vi "Main.vi"(10 "Productos Subpanel":refnum<vi>, 11 "Module Admin":refnum<class "Delacor_lib_QMH_Module Admin.lvclass">) -> ()   [LabVIEW 2020, in "Productos.lvlib"]
doc: "This template is based off of the Queued Message Handler design pattern and the Queued Message Handler project template that ships with LabVIEW.\n\nThe main difference is that the queue is private to this module and communication between modules is performed via Broadcast and Request events.\n\nRequest events are wrapped in public API methods and are handled in the Event Handling Loop (EHL) of this VI. Any module can register for Broadcast events sent by this module. The EHL generates messages based on user interface actions.\n\nThe Message Handling Loop (MHL) processes messages generated by the EHL, or by other messages. The messages are string values, so new messages can be added easily to the Message Cases case structure in the MHL. Each message cluster can also provide an optional value for Message Data, which is a variant that can be converted to whatever message-specific data is required.\n_____\nBased on Delacor QMH Project Template 5.0.0.82."
uses:
  Productos.lvlib
  <vilib>/Delacor/Delacor QMH/Libraries/Module Admin_class/Delacor_lib_QMH_Module Admin.lvclass
  Module Data--cluster.ctl
  Stop Argument--cluster.ctl
  <vilib>/Delacor/Delacor QMH/Libraries/Message Queue_class/Delacor_lib_QMH_Message Queue.lvclass/Delacor_lib_QMH_Message Queue.ctl
  <vilib>/Delacor/Delacor QMH/Libraries/Module Admin_class/Delacor_lib_QMH_Module Admin.lvclass/Delacor_lib_QMH_Module Admin.ctl
  <vilib>/Delacor/Delacor QMH/Libraries/Message Queue_class/Delacor_lib_QMH_Enqueue Message (Single).vi
  <vilib>/Delacor/Delacor QMH/Libraries/Module Admin_class/Delacor_lib_QMH_Get External Launch.vi
  <vilib>/Utility/error.llb/Error Cluster From Error Code.vi
  <vilib>/ErrorRing/Error Ring.xnode
  <vilib>/Delacor/Delacor QMH/Libraries/Message Queue_class/Delacor_lib_QMH_Message Queue.lvclass
panel:
  out "Status":string
  out "subarray":string[](array[string])
  in  "stop":bool
  in  "Products":i32(listbox)
  out "error out":errorcluster
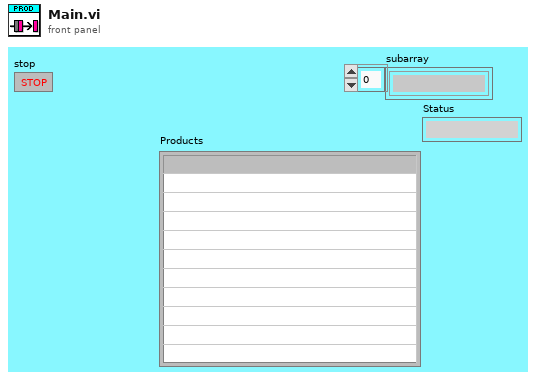
[diagram p1: front panel]
types:
  T1 = typedef "Productos.lvlib/Request Events--cluster.ctl" = cluster{"Stop Module":refnum<user-event>, "Show Panel":refnum<user-event>, "Hide Panel":refnum<user-event>, "Get Module Execution Status":refnum<user-event>, "Show Diagram":refnum<user-event>}
  T2 = typedef "Productos.lvlib/Module Data--cluster.ctl" = cluster{"Status":string}
  T3 = enum32{"invalid lock state", "Not Locked", "Locked (No Password)", "Password-protected"}
  T4 = typedef "Productos.lvlib/Stop Argument--cluster.ctl" = cluster{"Origin":string, "Exit via Stop Module Req?":bool, "Wait for Module to stop?":bool}
  T5 = enum32{"Invalid", "Standard", "Closed", "Hidden", "Minimized", "Maximized"}
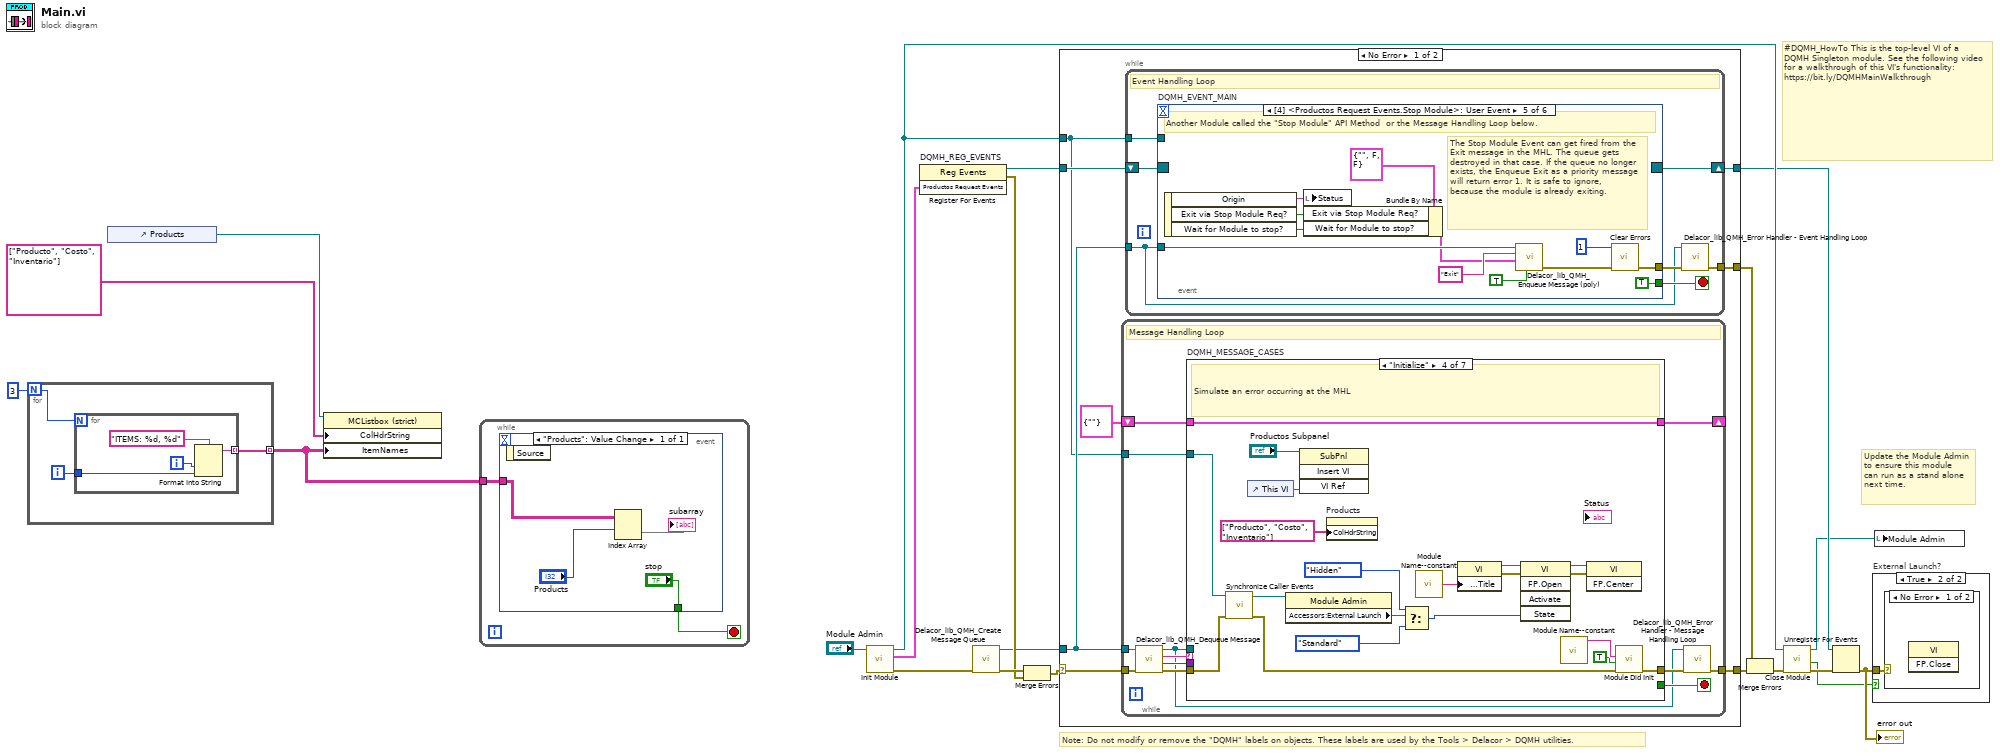
[diagram p0: block diagram]
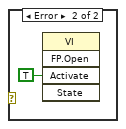
[diagram p3: hidden frame]
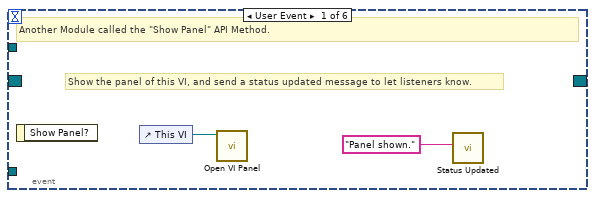
[diagram p4: hidden frame]
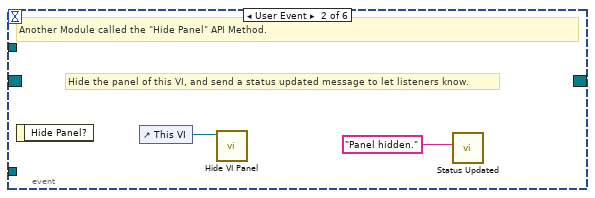
[diagram p5: hidden frame]
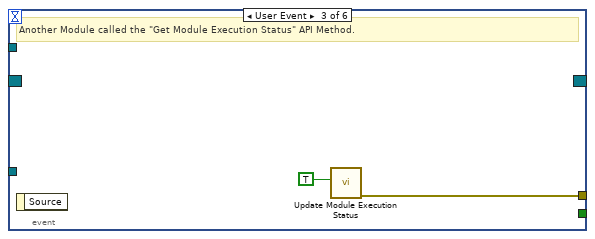
[diagram p6: hidden frame]
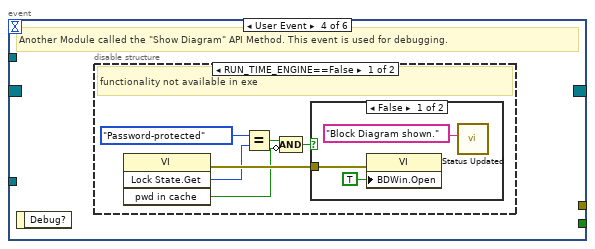
[diagram p7: hidden frame]
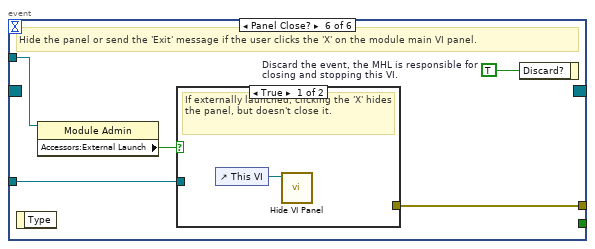
[diagram p10: hidden frame]
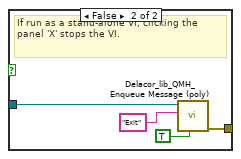
[diagram p11: hidden frame]
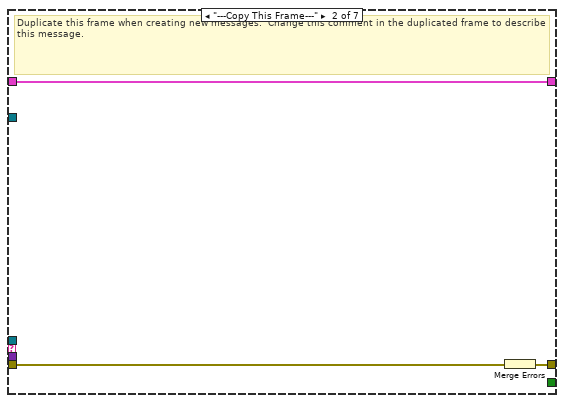
[diagram p13: hidden frame]
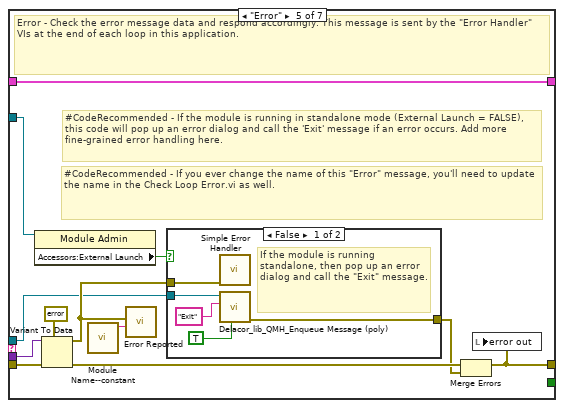
[diagram p15: hidden frame]
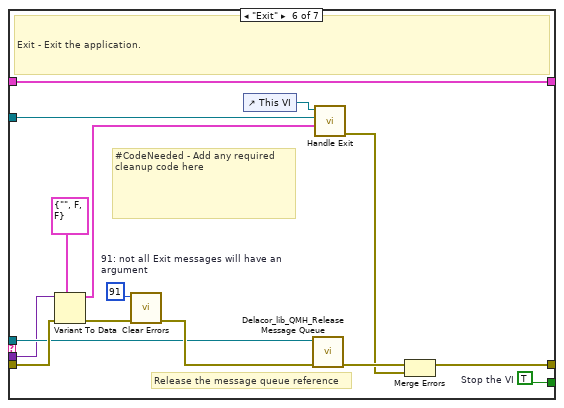
[diagram p17: hidden frame]
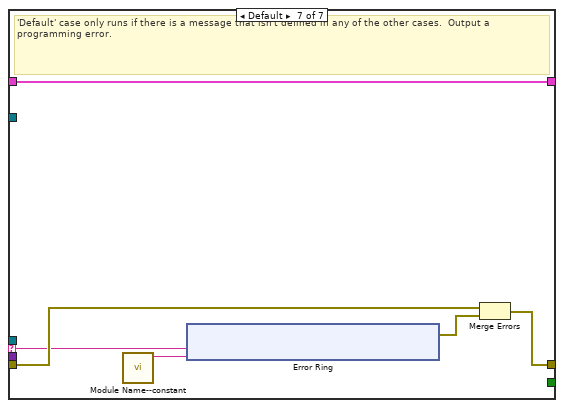
[diagram p18: hidden frame]
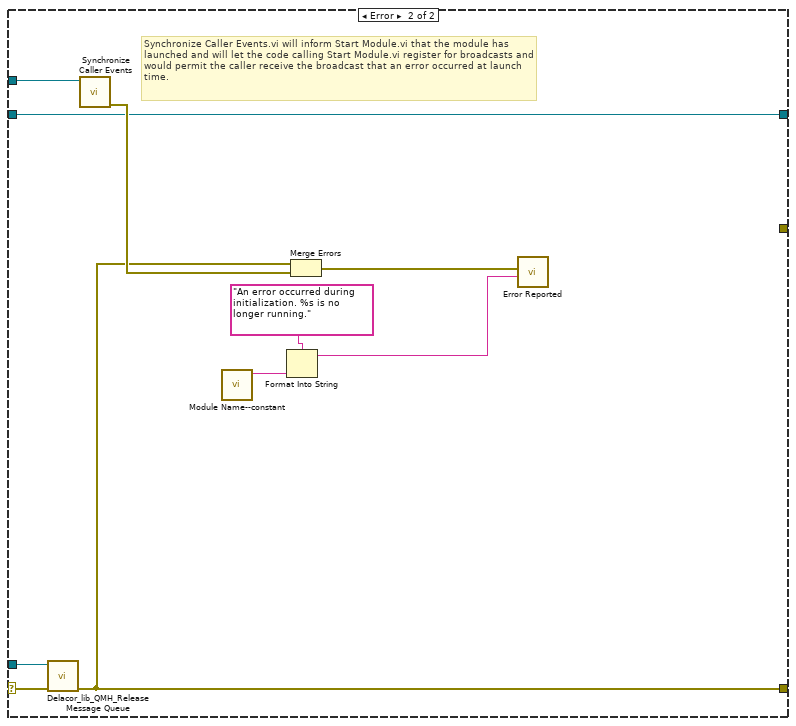
[diagram p19: hidden frame]
diagram:
  # "#DQMH_HowTo This is the top-level VI of a DQMH Singleton module. See the following video for a walkthrough of this VI's functionality: https://bit.ly/DQMHMainWalkthrough"
  # "Note: Do not modify or remove the \"DQMH\" labels on objects. These labels are used by the Tools > Delacor > DQMH utilities."
  # "Update the Module Admin to ensure this module can run as a stand alone next time."
  n1 = for {
    N: 3 -> [w24]
    tunnel: [w23] -> w1 mode=indexing
    i -> [w22]
    n2 = for {
      N: w24 -> [_]
      tunnel: [w27] -> w23 mode=indexing
      tunnel: w22 -> [w25]
      i -> [w28]
      n3 = Format Into String(format string="ITEMS: %d, %d", w28, w25) -> (resulting string=w27:string)  [unwired: 2 in, 1 out]
    }
  }
  n4 = control-ref of="Products"() -> (w4:refnum<vi>)
  n5 = property class="MCListbox (strict)"(reference=w4, "ColHdrString"=string[] ["Producto", "Costo", "Inventario"] ("Column Header Strings[]"), "ItemNames"=w1) -> ()  [unwired: 1 in, 2 out]
  n6 = while {
    tunnel: w1 -> [w30]
    stop <- w29 stop-if-true
    n7 = event shown="[0] \"Products\": Value Change" {
      selector: _ -> [_]
      dyn-events: _ -> [_]
      timeout: _ -> [_]
      tunnel: w30 -> [w34]
      tunnel: ["stop"] -> w29
      event "Products": Value Change {
        n8 = event-data() -> ()  [unwired: 1 in, 1 out]
        n9 = Index Array(array=w34, index (row)="Products") -> (element=→"subarray":string[])  [unwired: 1 in]
      }
    }
  }
  n10 = call "Init Module.vi"("Singleton Module Admin in"="Module Admin") -> ("error out"=w20:errorcluster, "Productos Request Events"=w9:T1, "Singleton Module Admin out"=w12:refnum<class "Delacor_lib_QMH_Module Admin.lvclass">)  [unwired: 8 in]
  n11 = register-events "DQMH_REG_EVENTS"(w9) -> (reference out=w10:refnum<event-registration>, error out=w13:errorcluster)  [unwired: 2 in]
  n12 = call <vilib>:"Delacor_lib_QMH_Create Message Queue.vi"("error in (no error)"=w20) -> ("error out"=w15:errorcluster, "Message Queue"=w8:refnum<class "Delacor_lib_QMH_Message Queue.lvclass">)  [unwired: 9 in]
  n13 = Merge Errors(w15, w13) -> (w14:errorcluster)
  n14 = case shown="No Error" w14 {
    selector: w14 -> [w40 w174]
    tunnel: [w42 w173] -> w21
    tunnel: [w39 w179] -> w11
    tunnel: w10 -> [w37 w179]
    tunnel: w8 -> [w36 w172]
    tunnel: [w41 _] -> w18
    tunnel: w12 -> [w35 w175]
    frame No Error {
      n15 = while {
        tunnel: w36 -> [w89]
        shift-right: [w93] -> _
        shift-left: T2 {"Status"=""} ("Data Cluster") -> [w94]
        tunnel: w40 -> [w97]
        tunnel: [w95] -> w42
        tunnel: w35 -> [w87]
        stop <- w92 stop-if-true
        # "Message Handling Loop"
        n16 = call-dynamic "Delacor_lib_QMH_Dequeue Message.vi"("error in (no error)"=w97, "Message Queue in"=w89) -> ("error out"=w96:errorcluster, "Message Data"=w90:variant, "Message"=w91:string, "Message Queue out"=w88:refnum<class "Delacor_lib_QMH_Message Queue.lvclass">)  [unwired: 6 in]
        n17 = case "DQMH_MESSAGE_CASES" shown="\"Initialize\"" w91 {
          selector: w91 -> [_ _ _ _ _ _ w159]
          tunnel: w88 -> [_ _ _ _ w129 w151 _]
          tunnel: w96 -> [w100 w103 w105 w124 w136 w157 w161]
          tunnel: [w100 w102 w105 w109 w132 w154 w162] -> w98
          tunnel: w94 -> [w99 w101 w104 w125 w131 w150 w160]
          tunnel: [w99 w101 w104 w125 w131 w150 w160] -> w93
          tunnel: [_ _ _ _ _ w149 _] -> w92
          tunnel: w90 -> [_ _ _ _ w130 w148 _]
          tunnel: w87 -> [_ _ _ w123 w128 w143 _]
          frame "--- Module Specific ---" {
            # "Separator -- The following cases handle messages specific to this Module."
          }
          frame "---Copy This Frame---" {
            # "Duplicate this frame when creating new messages.  Change this comment in the duplicated frame to describe this message."
            n18 = Merge Errors(w103) -> (w102:errorcluster)
          }
          frame "--- Exit and Error Handling---" {
            # "Separator - The following cases handle errors and exit messages."
          }
          frame "Initialize" {
            # "Simulate an error occurring at the MHL"
            n19 = call "Synchronize Caller Events.vi"("error in (no error)"=w124, "Singleton Module Admin in"=w123) -> ("error out"=w110:errorcluster, "Singleton Module Admin out"=w122:refnum<class "Delacor_lib_QMH_Module Admin.lvclass">)  [unwired: 8 in]
            n20 = control-ref of="This VI"() -> (w115:refnum<vi>)
            n21 = property class="Module Admin"(reference=w122) -> ("Accessors:External Launch"=w121:bool)  [unwired: 1 in, 2 out]
            n22 = invoke class="SubPnl" method="Insert VI"(reference="Productos Subpanel", "VI Ref"=w115) -> ()  [unwired: 2 in, 4 out]
            n23 = property on="Products" class="MCListbox (strict)"("ColHdrString"=string[] ["Producto", "Costo", "Inventario"] ("Column Header Strings[]")) -> ()  [unwired: 2 in, 2 out]
            n24 = Select(t=T5."Hidden" ("State"), s=w121, f=T5."Standard" ("State")) -> (s? t:f=w113:T5)
            n25 = call "Module Name--constant.vi"() -> ("Module Name"=w114:string)  [unwired: 11 in]
            n26 = property class="VI"("Front Panel.Title"=w114) -> (reference out=w118:refnum<vi>, error out=w120:errorcluster)  [unwired: 2 in]
            n27 = invoke class="VI" method="FP.Open"(reference=w118, error in=w120, "State"=w113) -> (reference out=w117:refnum<vi>, error out=w119:errorcluster)  [unwired: 2 in, 3 out]
            n28 = call "Module Name--constant.vi"() -> ("Module Name"=w108:string)  [unwired: 11 in]
            n29 = invoke class="VI" method="FP.Center"(reference=w117, error in=w119) -> ()  [unwired: 1 in, 3 out]
            n30 = call "Module Did Init.vi"("error in (no error)"=w110, "Initialized?"=TRUE, "Origin"=w108) -> ("error out"=w109:errorcluster)  [unwired: 8 in]
          }
          frame "Error" {
            # "#CodeRecommended - If you ever change the name of this \"Error\" message, you'll need to update the name in the Check Loop Error.vi as well."
            # "#CodeRecommended - If the module is running in standalone mode (External Launch = FALSE), this code will pop up an error dialog and call the 'Exit' message if an error occurs. Add more fine-grained error handling here."
            # "Error - Check the error message data and respond accordingly. This message is sent by the \"Error Handler\" VIs at the end of each loop in this application."
            n31 = property class="Module Admin"(reference=w128) -> ("Accessors:External Launch"=w127:bool)  [unwired: 1 in, 2 out]
            n32 = Variant To Data(error in=w136, type=errorcluster {"status"=FALSE, "code"=0, "source"=""} ("error constant"), Variant=w130) -> (data=w137:errorcluster, error out=w134:errorcluster)
            n33 = call "Module Name--constant.vi"() -> ("Module Name"=w126:string)  [unwired: 11 in]
            n34 = call "Error Reported.vi"("Additional Information"=w126, "Error"=w137) -> ()  [unwired: 9 in, 1 out]
            n35 = case shown="False" w127 {
              tunnel: [w142 _] -> w133
              tunnel: w129 -> [w140 _]
              tunnel: w137 -> [w141 _]
              frame False {
                # "If the module is running standalone, then pop up an error dialog and call the \"Exit\" message."
                n36 = call <vilib>:"Simple Error Handler.vi"("error in (no error)"=w141) -> ()  [unwired: 4 in, 5 out]
                n37 = call-poly <vilib>:"Delacor_lib_QMH_Enqueue Message (poly).vi"("Priority Message? (F)"=TRUE, "Message"="Exit", "Message Queue in"=w140) -> ("error out"=w142:errorcluster)  [unwired: 7 in, 1 out]
              }
              frame True {
                # "If the module was launched externally, calling the Error Reported broadcast VI is the only action performed by the \"Error\" message. The module's caller can then process the error appropriately."
              }
            }
            n38 = Merge Errors(w134, w133) -> (w132:errorcluster)
            n39 = local write "error out"(w132) -> ()
          }
          frame "Exit" {
            w147 = 91  # 91: not all Exit messages will have an argument
            w149 = TRUE  # Stop the VI
            # "Release the message queue reference"
            # "#CodeNeeded - Add any required cleanup code here"
            # "Exit - Exit the application."
            n40 = Variant To Data(error in=w157, type=T4 {"Origin"="", "Exit via Stop Module Req?"=FALSE, "Wait for Module to stop?"=FALSE} ("Stop Argument"), Variant=w148) -> (data=w145:T4, error out=w153:errorcluster)
            n41 = call <vilib>:"Clear Errors.vi"("error in (no error)"=w153, "specific error code to clear (0: all)"=w147) -> ("error out"=w156:errorcluster)  [unwired: 4 in, 1 out]
            n42 = control-ref of="This VI"() -> (w144:refnum<vi>)
            n43 = call-dynamic "Delacor_lib_QMH_Release Message Queue.vi"("error in (no error)"=w156, "Message Queue"=w151) -> ("error out"=w155:errorcluster)  [unwired: 9 in]
            n44 = call "Handle Exit.vi"("Stop Argument"=w145, "Admin in"=w143, "VI reference"=w144) -> ("error out"=w152:errorcluster)  [unwired: 7 in, 1 out]
            n45 = Merge Errors(w155, w152) -> (w154:errorcluster)
          }
          frame Default {
            # "'Default' case only runs if there is a message that isn't defined in any of the other cases.  Output a programming error."
            n46 = call "Module Name--constant.vi"() -> ("Module Name"=w158:string)  [unwired: 11 in]
            n47 = xnode "Error Ring"("parameter 0"=w159, "parameter 1"=w158) -> ("error out"=w163:errorcluster)
            n48 = Merge Errors(w161, w163) -> (w162:errorcluster)
          }
        }
        n49 = call-dynamic "Delacor_lib_QMH_Error Handler - Message Handling Loop.vi"("error in (no error)"=w98, "Message Queue in"=w88) -> ("dup error in"=w95:errorcluster)  [unwired: 8 in, 1 out]
      }
      n50 = while {
        tunnel: w36 -> [w43]
        shift-right: [w46] -> w39
        shift-left: w37 -> [w47]
        tunnel: [w48] -> w41
        tunnel: w35 -> [w44]
        stop <- w45 stop-if-true
        # "Event Handling Loop"
        n51 = event "DQMH_EVENT_MAIN" shown="[4] <Productos Request Events.Stop Module>: User Event" {
          selector: w47 -> [_ _ _ _ _ _]
          dyn-events: [_ _ _ _ _ _] -> w46
          timeout: _ -> [_ _ _ _ _ _]
          tunnel: [_ _ _ _ TRUE ("Discard?") _] -> w45
          tunnel: w43 -> [_ _ _ _ w72 w79]
          tunnel: [_ _ w55 _ w75 w81] -> w49
          tunnel: w44 -> [_ _ _ _ _ w78]
          event User Event {
            # "Show the panel of this VI, and send a status updated message to let listeners know."
            # "Another Module called the \"Show Panel\" API Method."
            n52 = event-data() -> ()  [unwired: 1 in, 1 out]
            n53 = control-ref of="This VI"() -> (w51:refnum<vi>)
            n54 = call "Open VI Panel.vi"("VI"=w51) -> ()  [unwired: 10 in, 1 out]
            n55 = call "Status Updated.vi"("Status"="Panel shown." ("format string")) -> ()  [unwired: 10 in, 1 out]
          }
          event User Event {
            # "Hide the panel of this VI, and send a status updated message to let listeners know."
            # "Another Module called the \"Hide Panel\" API Method."
            n56 = event-data() -> ()  [unwired: 1 in, 1 out]
            n57 = control-ref of="This VI"() -> (w53:refnum<vi>)
            n58 = call "Hide VI Panel.vi"("VI"=w53) -> ()  [unwired: 10 in, 1 out]
            n59 = call "Status Updated.vi"("Status"="Panel hidden." ("format string")) -> ()  [unwired: 10 in, 1 out]
          }
          event User Event {
            # "Another Module called the \"Get Module Execution Status\" API Method."
            n60 = event-data() -> ()  [unwired: 1 in, 1 out]
            n61 = call "Update Module Execution Status.vi"("Running?"=TRUE) -> ("error out"=w55:errorcluster)  [unwired: 10 in]
          }
          event User Event {
            # "Another Module called the \"Show Diagram\" API Method. This event is used for debugging."
            n62 = event-data() -> ()  [unwired: 1 in, 1 out]
            n63 = disable-structure shown="RUN_TIME_ENGINE==False" {
              frame condition #0 (active) {
                # "functionality not available in exe"
                n64 = invoke class="VI" method="Lock State.Get"() -> (error out=w61:errorcluster, "Get Lock State"=w60:T3, "pwd in cache"=w57:bool)  [unwired: 4 in, 1 out]
                n65 = Equal?(x=T3."Password-protected", y=w60) -> (x = y?=w58:bool)
                n66 = Compound Arithmetic op=AND(w58, invert w57) -> (w56:bool)
                n67 = case shown="False" w56 {
                  tunnel: w61 -> [w64 _]
                  frame False {
                    n68 = property class="VI"(error in=w64, "BDWin.Open"=TRUE ("Block Diagram Window:Open")) -> ()  [unwired: 1 in, 2 out]
                    n69 = call "Status Updated.vi"("Status"="Block Diagram shown." ("format string")) -> ()  [unwired: 10 in, 1 out]
                  }
                  frame True {
                    # "Password-protected VI, and the password is not in the cache. Do not show the diagram."
                  }
                }
              }
              frame condition #1 {
              }
            }
          }
          event User Event {
            # "The Stop Module Event can get fired from the Exit message in the MHL. The queue gets destroyed in that case. If the queue no longer exists, the Enqueue Exit as a priority message will return error 1. It is safe to ignore, because the module is already exiting."
            # "Another Module called the \"Stop Module\" API Method  or the Message Handling Loop below."
            n70 = event-data() -> ("Origin"=w65:string, "Exit via Stop Module Req?"=w68:bool, "Wait for Module to stop?"=w67:bool)  [unwired: 1 in]
            n71 = local write "Status"(w65) -> ()
            n72 = Bundle By Name(cluster=T4 {"Origin"="", "Exit via Stop Module Req?"=FALSE, "Wait for Module to stop?"=FALSE} ("Stop Argument"), "Exit via Stop Module Req?"=w68, "Wait for Module to stop?"=w67) -> (w66:T4)
            n73 = call-poly <vilib>:"Delacor_lib_QMH_Enqueue Message (poly).vi"("Priority Message? (F)"=TRUE, "Message Data"=w66, "Message"="Exit", "Message Queue in"=w72) -> ("error out"=w76:errorcluster)  [unwired: 6 in, 1 out]
            n74 = call <vilib>:"Clear Errors.vi"("error in (no error)"=w76, "specific error code to clear (0: all)"=1) -> ("error out"=w75:errorcluster)  [unwired: 4 in, 1 out]
          }
          event Panel Close? {
            w80 = TRUE  # Discard the event, the MHL is responsible for closing and stopping this VI.
            # "Hide the panel or send the 'Exit' message if the user clicks the 'X' on the module main VI panel."
            n75 = event-data() -> ()  [unwired: 1 in, 1 out]
            n76 = property class="Module Admin"(reference=w78) -> ("Accessors:External Launch"=w77:bool)  [unwired: 1 in, 2 out]
            n77 = case shown="True" w77 {
              tunnel: w79 -> [_ w85]
              tunnel: [_ w86] -> w81
              frame True {
                # "If externally launched, clicking the 'X' hides the panel, but doesn't close it."
                n78 = control-ref of="This VI"() -> (w82:refnum<vi>)
                n79 = call "Hide VI Panel.vi"("VI"=w82) -> ()  [unwired: 10 in, 1 out]
              }
              frame False {
                # "If run as a stand-alone VI, clicking the panel 'X' stops the VI."
                n80 = call-poly <vilib>:"Delacor_lib_QMH_Enqueue Message (poly).vi"("Priority Message? (F)"=TRUE, "Message"="Exit", "Message Queue in"=w85) -> ("error out"=w86:errorcluster)  [unwired: 7 in, 1 out]
              }
            }
            n81 = event-data("Discard?"=w80) -> ()  [unwired: 1 in, 1 out]
          }
        }
        n82 = call-dynamic "Delacor_lib_QMH_Error Handler - Event Handling Loop.vi"("error in (no error)"=w49, "Message Queue in"=w43) -> ("dup error in"=w48:errorcluster)  [unwired: 8 in, 1 out]
      }
    }
    frame Error {
      # "Synchronize Caller Events.vi will inform Start Module.vi that the module has launched and will let the code calling Start Module.vi register for broadcasts and would permit the caller receive the broadcast that an error occurred at launch time."
      n83 = call-dynamic "Delacor_lib_QMH_Release Message Queue.vi"("error in (no error)"=w174, "Message Queue"=w172) -> ("error out"=w173:errorcluster)  [unwired: 9 in]
      n84 = call "Synchronize Caller Events.vi"("Singleton Module Admin in"=w175) -> ("error out"=w180:errorcluster)  [unwired: 9 in, 1 out]
      n85 = call "Module Name--constant.vi"() -> ("Module Name"=w178:string)  [unwired: 11 in]
      n86 = Format Into String(format string="An error occurred during initialization. %s is no longer running.", w178) -> (resulting string=w176:string)  [unwired: 2 in, 1 out]
      n87 = Merge Errors(w173, w180) -> (w181:errorcluster)
      n88 = call "Error Reported.vi"("Additional Information"=w176, "Error"=w181) -> ()  [unwired: 9 in, 1 out]
    }
  }
  n89 = Merge Errors(w18, w21) -> (w17:errorcluster)
  n90 = call "Close Module.vi"("error in (no error)"=w17, "Module Admin in"=w12) -> ("error out"=w19:errorcluster, "External Launch"=w5:bool, "Module Admin out"=w6:refnum<class "Delacor_lib_QMH_Module Admin.lvclass">)  [unwired: 7 in]
  n91 = Unregister For Events(event registration refnum=w11, error in=w19) -> (error out=w16:errorcluster)
  "error out" <- w16
  n92 = case "External Launch?" shown="True" w5 {
    tunnel: w16 -> [_ w182]
    frame False {
    }
    frame True {
      n93 = case shown="No Error" w182 {
        frame No Error {
          n94 = invoke class="VI" method="FP.Close"() -> ()  [unwired: 3 in, 3 out]
        }
        frame Error {
          n95 = invoke class="VI" method="FP.Open"("Activate"=TRUE ("Activate?")) -> ()  [unwired: 4 in, 5 out]
        }
      }
    }
  }
  n96 = local write "Module Admin"(w6) -> ()
